vi "IMUOrientOpenWithRST.vi"() -> ()   [LabVIEW 2015]
uses:
  <vilib>/Rock Robotics/SystemInterfaces/i2clib/i2c_bus.ctl
  <vilib>/Rock Robotics/SystemInterfaces/DIO/FPGA_DIOChannel.ctl
  <vilib>/Rock Robotics/WPI/I2C/WPI_I2CDevRef.ctl
panel:
  out "Bad result":bool
  out "Fatal Result":bool
  out "Cal Status":T1
  out "I2CDevRef":T2={"DevStatus"={"status"=FALSE, "code"=0, "source"=""}, "Device Address"=0, "Handle"=0, "I2C Bus"=enum."Invalid"} {"Device Address" format="%.0x"}
  in  "DIO Channel":T4
  in  "Stored Cal File":string="BNO055 Cal MC P3 11-28-2015 145653"
  in  "Calibrate?":bool
  in  "Status delay":i32=30
  in  "I2C Bus":T3=enum."I2C MXP"
  in  "Placement":T5(ring)=enum."P3"
  in  "Op Mode":T6(ring)=enum."NDOF"
  # "Manual Cal\nCalibration Status Indicator"
  # "Diagnostics"
  # "These controls/indicators are non-operational / they are here as example documentation only."
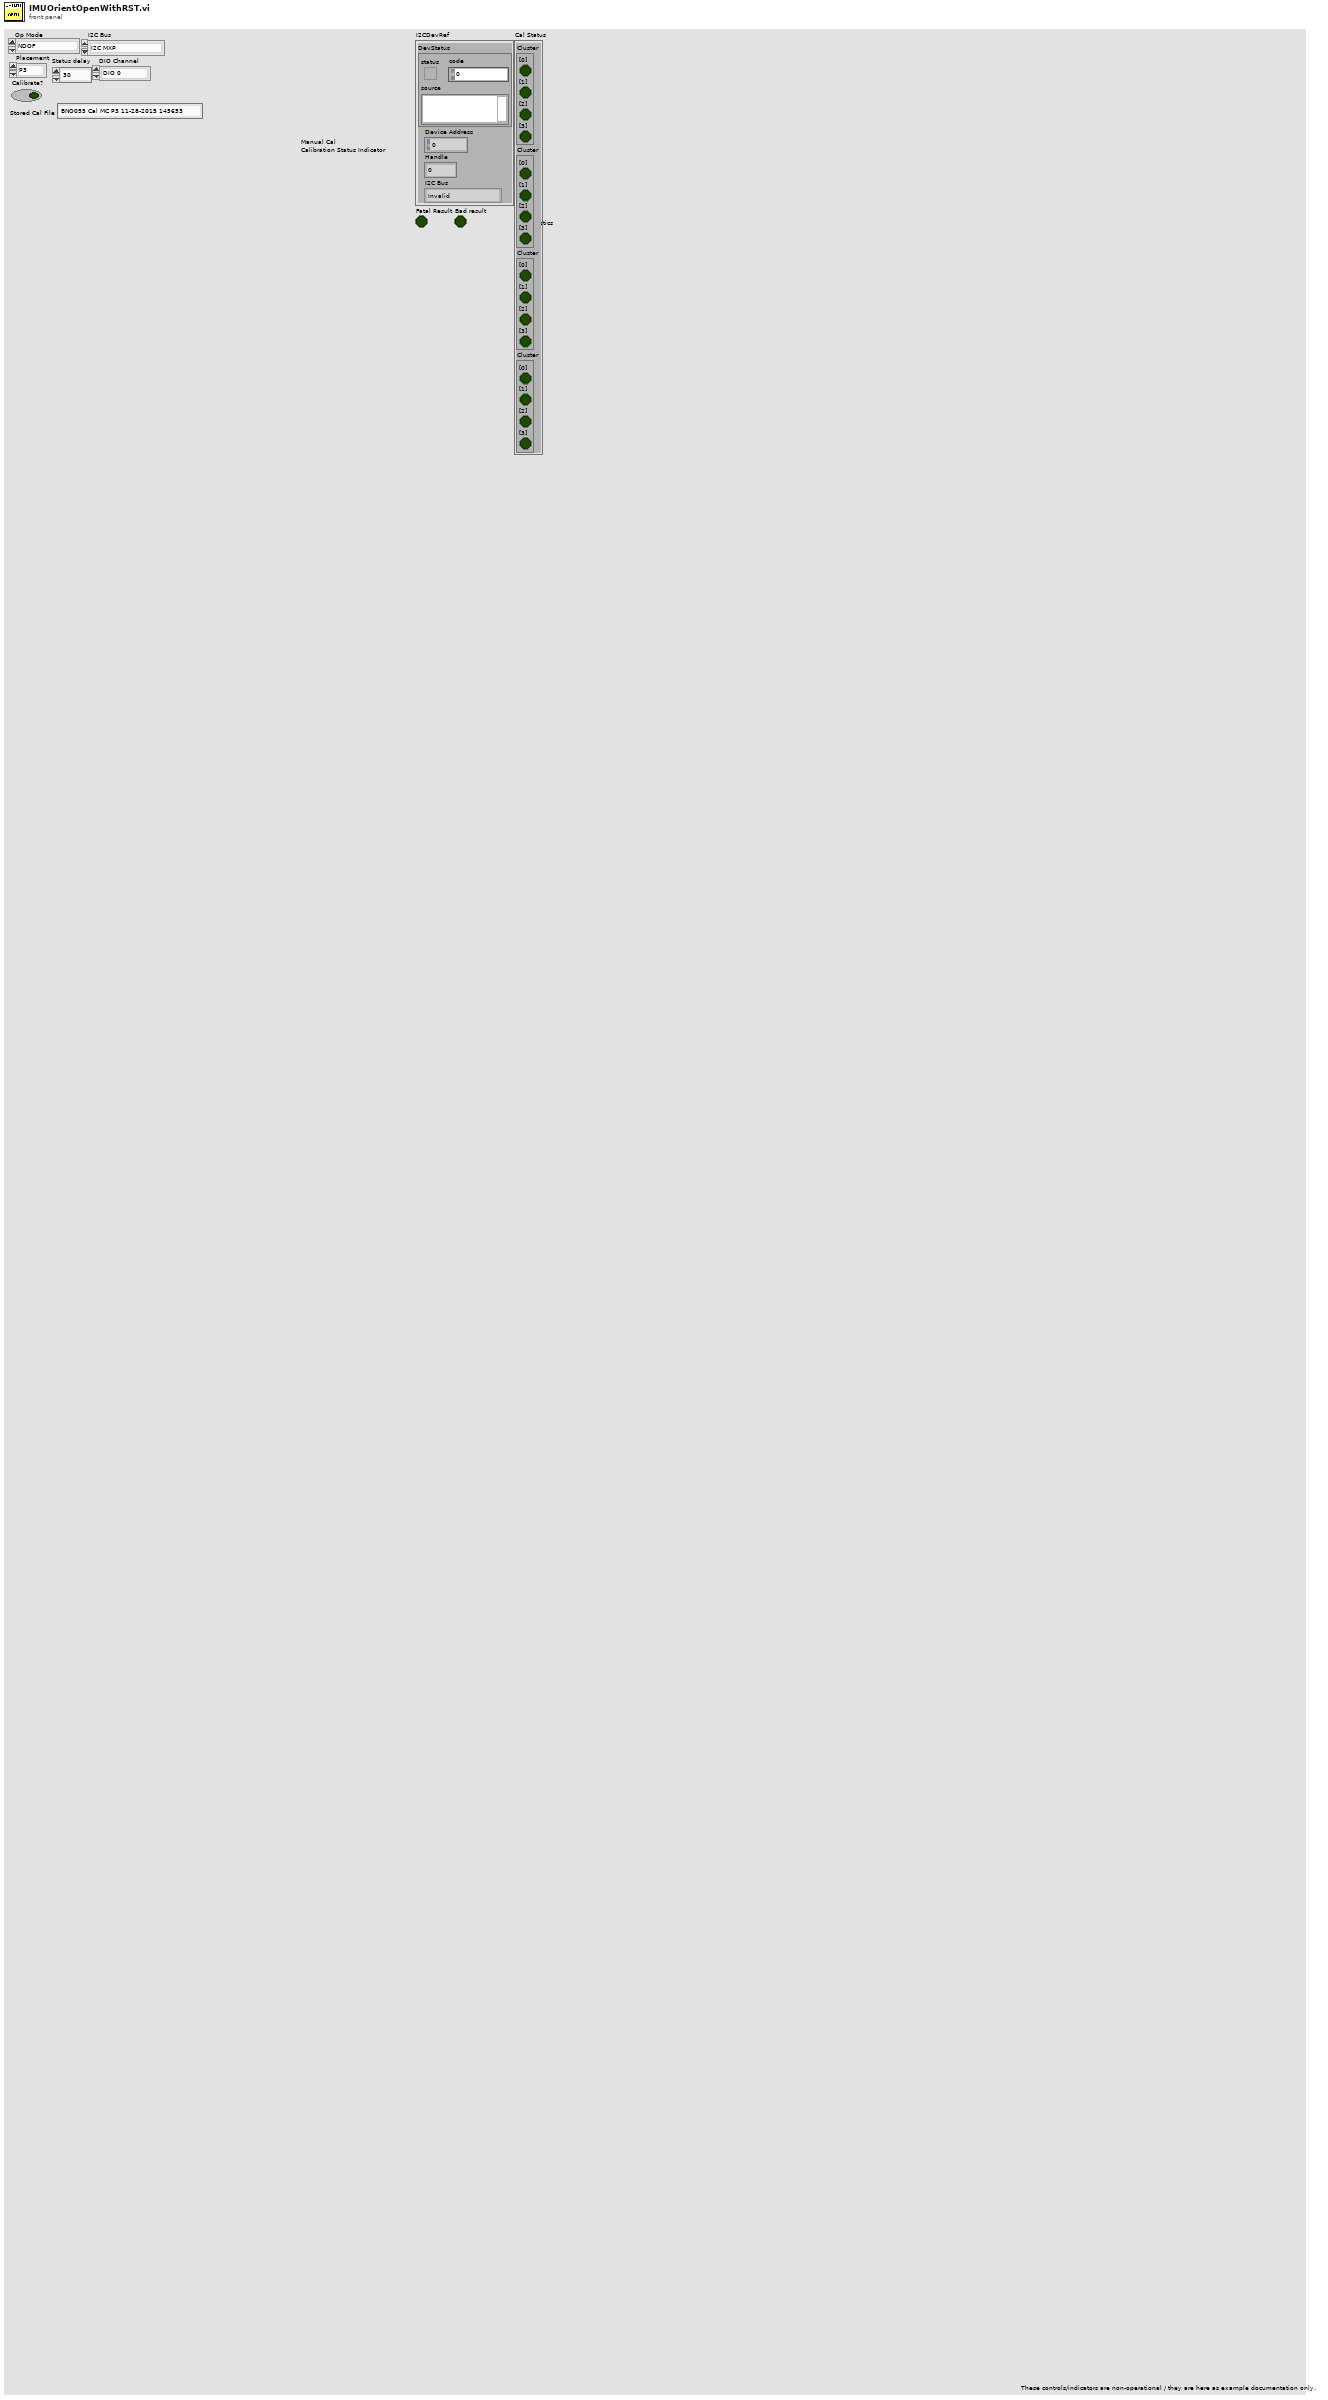
[diagram p1: front panel]
types:
  T1 = cluster{"Cluster":cluster{"[0]":bool, "[1]":bool, "[2]":bool, "[3]":bool}, "Cluster":cluster{"[0]":bool, "[1]":bool, "[2]":bool, "[3]":bool}, "Cluster":cluster{"[0]":bool, "[1]":bool, "[2]":bool, "[3]":bool}, "Cluster":cluster{"[0]":bool, "[1]":bool, "[2]":bool, "[3]":bool}}
  T2 = typedef "WPI_I2CDevRef.ctl" = cluster{"DevStatus":errorcluster, "Device Address":u8, "Handle":i32, "I2C Bus":T3}
  T3 = typedef "i2c_bus.ctl" = enum16{"I2C On-Board", "I2C MXP", "Invalid"}
  T4 = typedef "FPGA_DIOChannel.ctl" = enum8{"DIO 0", "DIO 1", "DIO 2", "DIO 3", "DIO 4", "DIO 5", "DIO 6", "DIO 7", "DIO 8", "DIO 9", "DIO MXP 0", "DIO MXP 1", "DIO MXP 2", "DIO MXP 3", "DIO MXP 4", "DIO MXP 5", "DIO MXP 6", "DIO MXP 7", "DIO MXP 8", "DIO MXP 9", "DIO MXP 10", "DIO MXP 11", "DIO MXP 12", "DIO MXP 13", "DIO MXP 14", "DIO MXP 15", "Invalid"}
  T5 = enum32{"P0", "P1", "P2", "P3", "P4", "P5", "P6", "P7"}
  T6 = enum8{"ConfigMode", "AccOnly", "MagOnly", "GyroOnly", "AccMag", "AccGyro", "MagGyro", "AMG", "IMU", "Compass", "M4G", "NDOF_FMC_OFF", "NDOF"}
  T7 = typedef "WPI_DigitalOutputDevRef.ctl" = cluster{"DIO Channel":T4, "DevStatus":errorcluster}
  T8 = cluster{"Op Mode":enum8{"ConfigMode", "AccOnly", "MagOnly", "GyroOnly", "AccMag", "AccGyro", "MagGyro", "AMG", "IMU", "Compass", "M4G", "NDOF_FMC_OFF", "NDOF"}, "Placement":enum32{"P0", "P1", "P2", "P3", "P4", "P5", "P6", "P7"}, "I2C Bus":T3, "Status delay":i32}
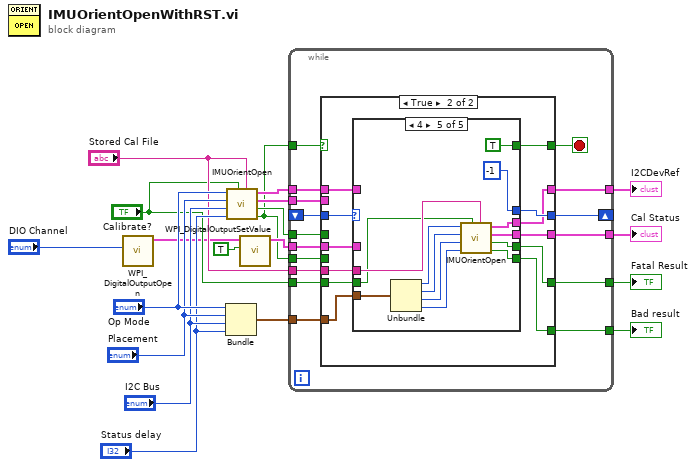
[diagram p0: block diagram]
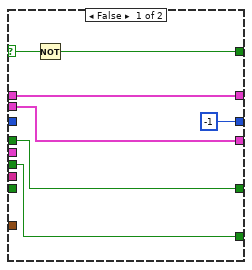
[diagram p2: hidden frame]
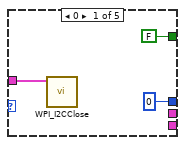
[diagram p3: hidden frame]
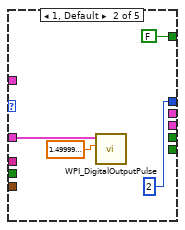
[diagram p4: hidden frame]
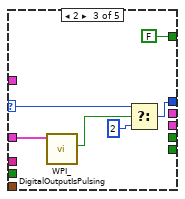
[diagram p5: hidden frame]
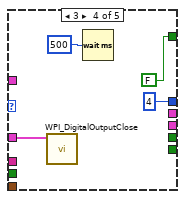
[diagram p6: hidden frame]
diagram:
  n1 = call <vilib>:"WPI_DigitalOutputOpen.vi"("DIO Channel"="DIO Channel") -> ("DigitalOutputDevRef"=w4:T7)  [unwired: 9 in, 1 out]
  n2 = Bundle("Op Mode"="Op Mode", "Placement"="Placement", "I2C Bus"="I2C Bus", "Status delay"="Status delay") -> (w13:T8)  [unwired: 1 in]
  n3 = call "IMUOrientOpen.vi"("Stored Cal File"="Stored Cal File", "Calibrate?"="Calibrate?", "Status delay"="Status delay", "I2C Bus"="I2C Bus", "Placement"="Placement", "Op Mode"="Op Mode") -> ("Bad result"=w1:bool, "Fatal Result"=w10:bool, "Cal Status"=w11:T1, "I2CDevRef"=w19:T2)  [unwired: 1 in, 1 out]
  n4 = call <vilib>:"WPI_DigitalOutputSetValue.vi"("Value"=TRUE, "DigitalOutputDevRef"=w4) -> ("DigitalOutputDevRef"=w2:T7)  [unwired: 8 in, 1 out]
  n5 = while {
    tunnel: w1 -> [w30]
    tunnel: w19 -> [w35]
    shift-right: [w34] -> _
    shift-left: _ -> [w33]
    tunnel: w2 -> [w32]
    tunnel: w13 -> [w31]
    tunnel: "Stored Cal File" -> [w28]
    tunnel: [w27] -> w9
    tunnel: w11 -> [w26]
    tunnel: [w25] -> w8
    tunnel: [w24] -> w7
    tunnel: w10 -> [w23]
    tunnel: w1 -> [w22]
    tunnel: [w21] -> w6
    tunnel: "Calibrate?" -> [w20]
    stop <- w29 stop-if-true
    n6 = case shown="True" w30 {
      selector: w30 -> [w40 _]
      tunnel: w35 -> [w39 w43]
      tunnel: [-1 ("f") w53] -> w34
      tunnel: w33 -> [_ w54]
      tunnel: w32 -> [_ w52]
      tunnel: w31 -> [_ w51]
      tunnel: [w41 w50] -> w29
      tunnel: w28 -> [_ w49]
      tunnel: [w39 w48] -> w27
      tunnel: [w38 w47] -> w25
      tunnel: w26 -> [w38 _]
      tunnel: [w37 w46] -> w24
      tunnel: w23 -> [w37 _]
      tunnel: [w36 w45] -> w21
      tunnel: w22 -> [w36 _]
      tunnel: w20 -> [_ w44]
      frame False {
        n7 = Not(x=w40) -> (.not. x?=w41:bool)
      }
      frame True {
        n8 = case shown="4" w54 {
          selector: w54 -> [_ _ w64 _ _]
          tunnel: [0 ("f") 2 ("f") w63 4 ("f") -1 ("f")] -> w53
          tunnel: w52 -> [_ w61 w65 w68 _]
          tunnel: w51 -> [_ _ _ _ w84]
          tunnel: [FALSE FALSE FALSE FALSE TRUE] -> w50
          tunnel: w49 -> [_ _ _ _ w78]
          tunnel: [_ _ _ _ w77] -> w48
          tunnel: [_ _ _ _ w76] -> w47
          tunnel: [_ _ _ _ w74] -> w46
          tunnel: [_ _ _ _ w73] -> w45
          tunnel: w44 -> [_ _ _ _ w72]
          tunnel: w43 -> [w57 _ _ _ _]
          frame 0 {
            n9 = call <vilib>:"WPI_I2CClose.vi"("I2CDevRef"=w57) -> ()  [unwired: 10 in, 1 out]
          }
          frame 1, Default {
            n10 = call <vilib>:"WPI_DigitalOutputPulse.vi"("length (Sec)"=sgl 1.5e-05, "DigitalOutputDevRef"=w61) -> ()  [unwired: 8 in, 2 out]
          }
          frame 2 {
            n11 = call <vilib>:"WPI_DigitalOutputIsPulsing.vi"("DigitalOutputDevRef"=w65) -> ("IsPulsing?"=w67:bool)  [unwired: 8 in, 2 out]
            n12 = Select(t=w64, s=w67, f=2) -> (s? t:f=w63:i32)
          }
          frame 3 {
            n13 = call <vilib>:"WPI_DigitalOutputClose.vi"("DigitalOutputDevRef"=w68) -> ()  [unwired: 10 in, 1 out]
            n14 = Wait (ms)(milliseconds to wait=u32 500) -> ()  [unwired: 1 out]
          }
          frame 4 {
            n15 = Unbundle(w84) -> ("Op Mode"=w83:T6, "Placement"=w82:T5, "I2C Bus"=w81:T3, "Status delay"=w80:i32)
            n16 = call "IMUOrientOpen.vi"("Stored Cal File"=w78, "Calibrate?"=w72, "Status delay"=w80, "I2C Bus"=w81, "Placement"=w82, "Op Mode"=w83) -> ("Bad result"=w73:bool, "Fatal Result"=w74:bool, "Cal Status"=w76:T1, "I2CDevRef"=w77:T2)  [unwired: 1 in, 1 out]
          }
        }
      }
    }
  }
  "I2CDevRef" <- w9
  "Cal Status" <- w8
  "Fatal Result" <- w7
  "Bad result" <- w6
